vi "Neutral_voltage_conversions.vi"(8 "Constant":dbl, 9 "Final Value":dbl, 10 "Initial value":dbl, 11 "Conversion":T1=enum."B Field Grad (G/cm)") -> (1 "Final Voltage":dbl, 2 "Initial voltage":dbl)   [LabVIEW 2016]
uses:
  Neutral_voltage_conversion_control.ctl
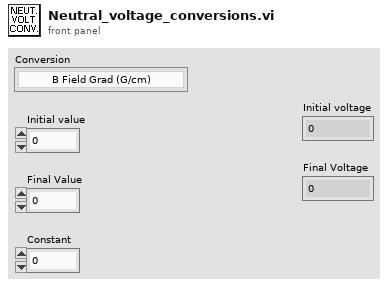
[diagram p1: front panel]
types:
  T1 = typedef "Neutral_voltage_conversion_control.ctl" = enum16{"Volts", "B Field Grad (G/cm)", "Red Boson Cntr Freq (MHz)", "Red Boson Dither Amp (kHz)", "Red Boson Power (mW)", "Red 87 Trap Cntr Freq (MHz)", "Red 87 Trap Dither Amp (kHz)", "Red 87 Trap Power (mW)", "Red 87 Stir Cntr Freq (MHz)", "Red 87 Stir Dither Amp (kHz)", "Red 87 Stir Power (mW)", "ODT Sheet Trap Power (W)", "ODT Loading Trap Power (W)"}
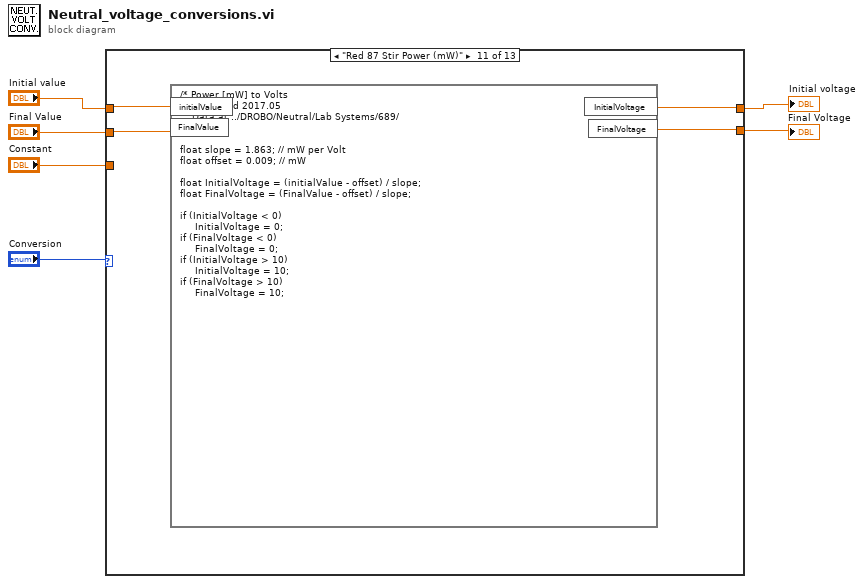
[diagram p0: block diagram]
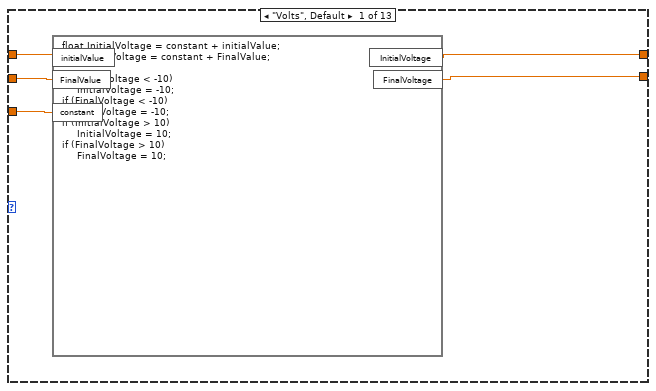
[diagram p2: hidden frame]
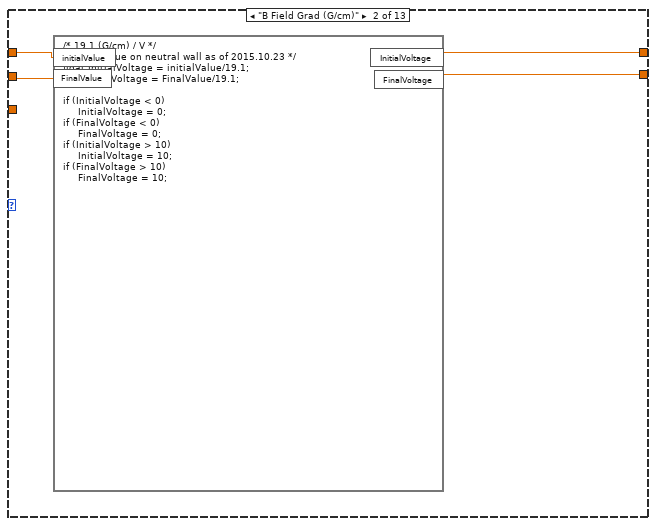
[diagram p3: hidden frame]
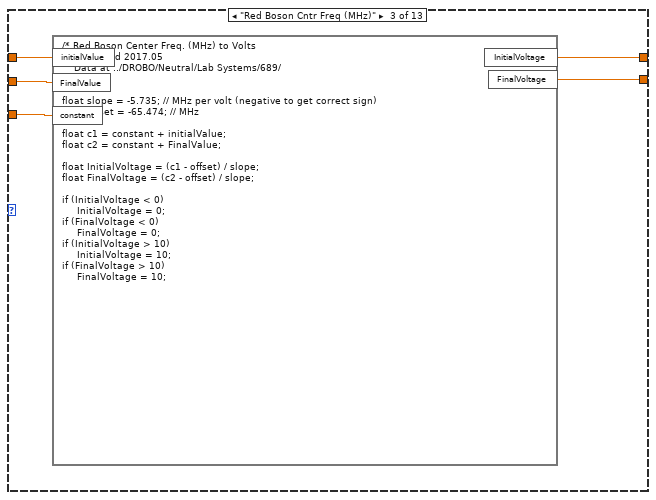
[diagram p4: hidden frame]
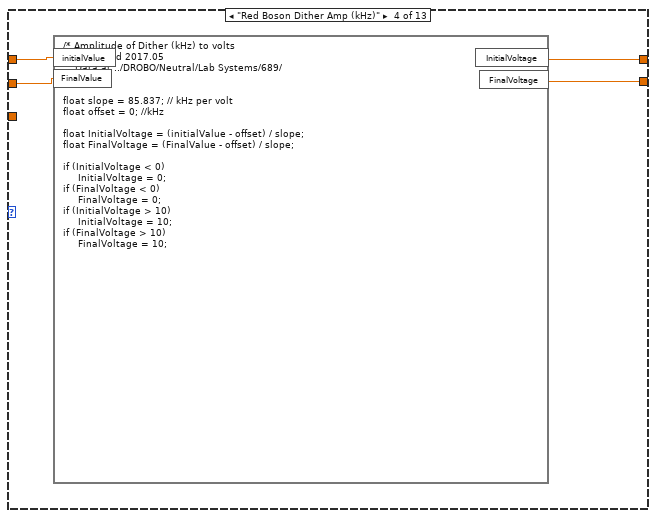
[diagram p5: hidden frame]
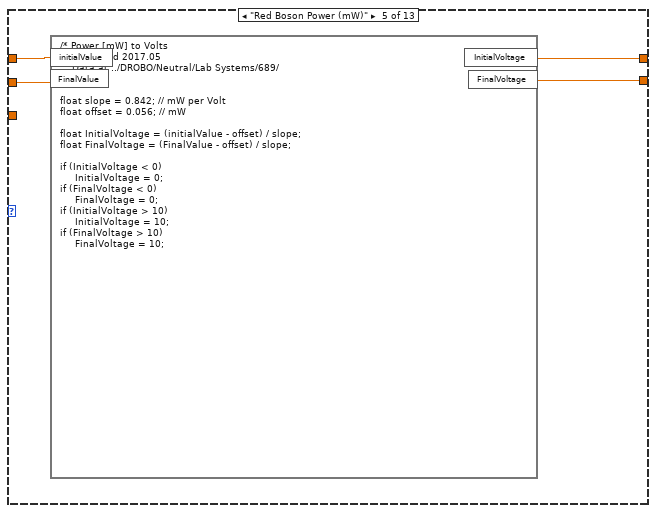
[diagram p6: hidden frame]
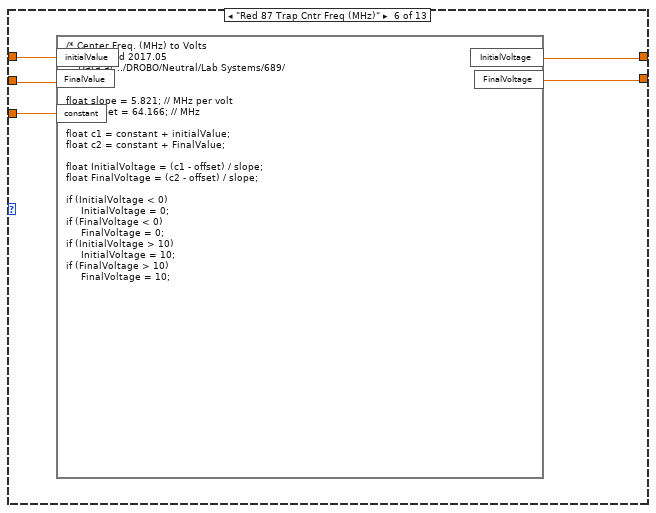
[diagram p7: hidden frame]
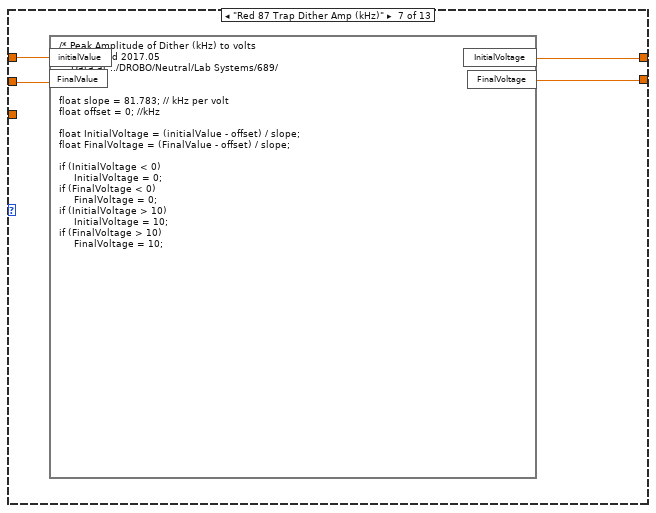
[diagram p8: hidden frame]
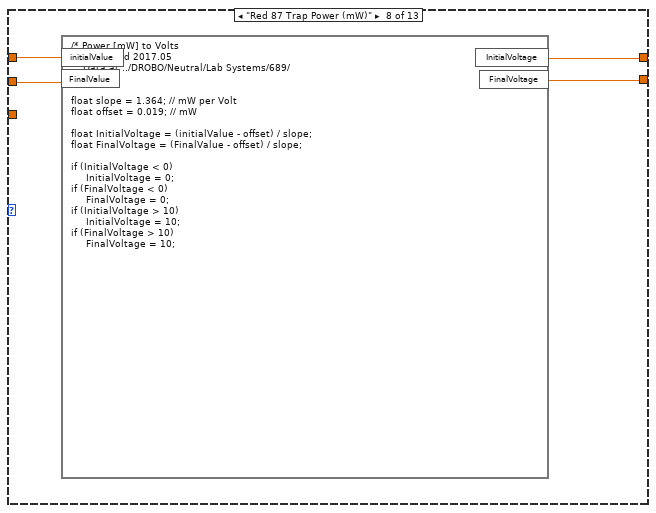
[diagram p9: hidden frame]
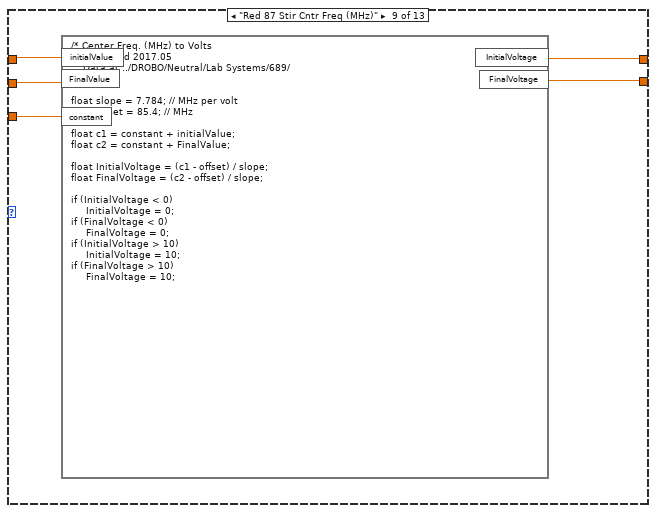
[diagram p10: hidden frame]
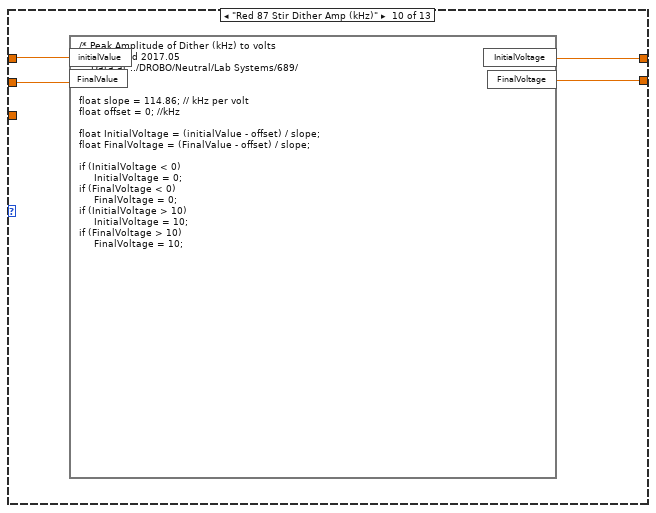
[diagram p11: hidden frame]
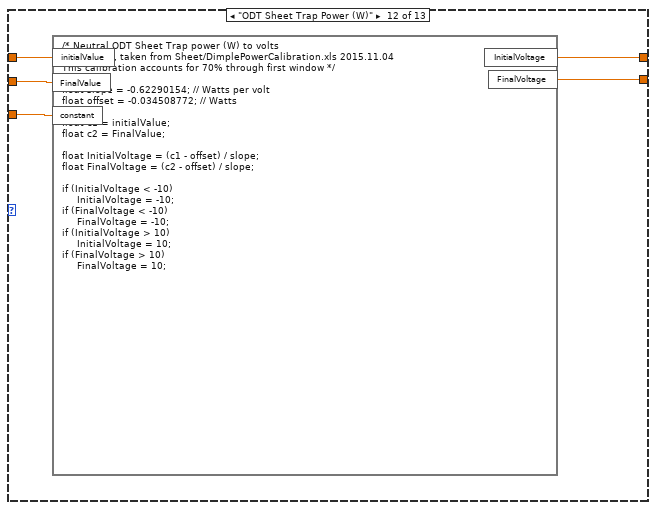
[diagram p12: hidden frame]
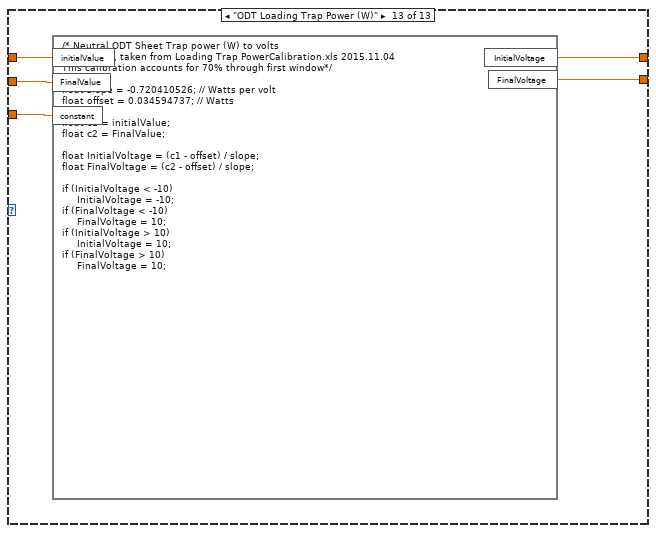
[diagram p13: hidden frame]
diagram:
  n1 = case shown="\"Red 87 Stir Power (mW)\"" "Conversion" {
    tunnel: "Initial value" -> [w9 w12 w20 w21 w28 w33 w35 w41 w46 w50 w54 w59 w64]
    tunnel: "Final Value" -> [w8 w13 w19 w22 w27 w32 w34 w40 w45 w49 w53 w58 w63]
    tunnel: [w10 w15 w18 w23 w25 w31 w36 w39 w43 w47 w52 w57 w62] -> w3
    tunnel: [w11 w14 w17 w24 w26 w30 w37 w38 w44 w48 w51 w56 w61] -> w2
    tunnel: "Constant" -> [w7 _ w16 _ _ w29 _ _ w42 _ _ w55 w60]
    frame "Volts", Default {
      n2 = formula code="float InitialVoltage = constant + initialValue;\nfloat FinalVoltage = constant + FinalValue;\n\nif (InitialVoltage < -10)\n     InitialVoltage = -10;\nif (FinalVoltage < -10)\n     FinalVoltage = -10;\nif (InitialVoltage > 10)\n     InitialVoltage = 10;\nif (FinalVoltage > 10)\n     FinalVoltage = 10;"("initialValue"=w9, "FinalValue"=w8, "constant"=w7) -> ("InitialVoltage"=w10:dbl, "FinalVoltage"=w11:dbl)
    }
    frame "B Field Grad (G/cm)" {
      n3 = formula code="/* 19.1 (G/cm) / V */\n/*Using value on neutral wall as of 2015.10.23 */\nfloat InitialVoltage = initialValue/19.1;\nfloat FinalVoltage = FinalValue/19.1;\n\nif (InitialVoltage < 0)\n     InitialVoltage = 0;\nif (FinalVoltage < 0)\n     FinalVoltage = 0;\nif (InitialVoltage > 10)\n     InitialVoltage = 10;\nif (FinalVoltage > 10)\n     FinalVoltage = 10;"("initialValue"=w12, "FinalValue"=w13) -> ("InitialVoltage"=w15:dbl, "FinalVoltage"=w14:dbl)
    }
    frame "Red Boson Cntr Freq (MHz)" {
      n4 = formula code="/* Red Boson Center Freq. (MHz) to Volts\n    Measured 2017.05\n    Data at ../DROBO/Neutral/Lab Systems/689/\n*/\n\nfloat slope = -5.735; // MHz per volt (negative to get correct sign)\nfloat offset = -65.474; // MHz\n\nfloat c1 = constant + initialValue;\nfloat c2 = constant + FinalValue;\n\nfloat InitialVoltage = (c1 - offset) / slope;\nfloat FinalVoltage = (c2 - offset) / slope;\n\nif (InitialVoltage < 0)\n     InitialVoltage = 0;\nif (FinalVoltage < 0)\n     FinalVoltage = 0;\nif (InitialVoltage > 10)\n     InitialVoltage = 10;\nif (FinalVoltage > 10)\n     FinalVoltage = 10;"("initialValue"=w20, "FinalValue"=w19, "constant"=w16) -> ("InitialVoltage"=w18:dbl, "FinalVoltage"=w17:dbl)
    }
    frame "Red Boson Dither Amp (kHz)" {
      n5 = formula code="/* Amplitude of Dither (kHz) to volts\n    Measured 2017.05\n    Data at ../DROBO/Neutral/Lab Systems/689/\n*/\n\nfloat slope = 85.837; // kHz per volt\nfloat offset = 0; //kHz\n\nfloat InitialVoltage = (initialValue - offset) / slope;\nfloat FinalVoltage = (FinalValue - offset) / slope;\n\nif (InitialVoltage < 0)\n     InitialVoltage = 0;\nif (FinalVoltage < 0)\n     FinalVoltage = 0;\nif (InitialVoltage > 10)\n     InitialVoltage = 10;\nif (FinalVoltage > 10)\n     FinalVoltage = 10;"("initialValue"=w21, "FinalValue"=w22) -> ("InitialVoltage"=w23:dbl, "FinalVoltage"=w24:dbl)
    }
    frame "Red Boson Power (mW)" {
      n6 = formula code="/* Power [mW] to Volts\n    Measured 2017.05\n    Data at ../DROBO/Neutral/Lab Systems/689/\n*/\n\nfloat slope = 0.842; // mW per Volt\nfloat offset = 0.056; // mW\n\nfloat InitialVoltage = (initialValue - offset) / slope;\nfloat FinalVoltage = (FinalValue - offset) / slope;\n\nif (InitialVoltage < 0)\n     InitialVoltage = 0;\nif (FinalVoltage < 0)\n     FinalVoltage = 0;\nif (InitialVoltage > 10)\n     InitialVoltage = 10;\nif (FinalVoltage > 10)\n     FinalVoltage = 10;"("initialValue"=w28, "FinalValue"=w27) -> ("InitialVoltage"=w25:dbl, "FinalVoltage"=w26:dbl)
    }
    frame "Red 87 Trap Cntr Freq (MHz)" {
      n7 = formula code="/* Center Freq. (MHz) to Volts\n    Measured 2017.05\n    Data at ../DROBO/Neutral/Lab Systems/689/\n*/\n\nfloat slope = 5.821; // MHz per volt\nfloat offset = 64.166; // MHz\n\nfloat c1 = constant + initialValue;\nfloat c2 = constant + FinalValue;\n\nfloat InitialVoltage = (c1 - offset) / slope;\nfloat FinalVoltage = (c2 - offset) / slope;\n\nif (InitialVoltage < 0)\n     InitialVoltage = 0;\nif (FinalVoltage < 0)\n     FinalVoltage = 0;\nif (InitialVoltage > 10)\n     InitialVoltage = 10;\nif (FinalVoltage > 10)\n     FinalVoltage = 10;"("initialValue"=w33, "FinalValue"=w32, "constant"=w29) -> ("InitialVoltage"=w31:dbl, "FinalVoltage"=w30:dbl)
    }
    frame "Red 87 Trap Dither Amp (kHz)" {
      n8 = formula code="/* Peak Amplitude of Dither (kHz) to volts\n    Measured 2017.05\n    Data at ../DROBO/Neutral/Lab Systems/689/\n*/\n\nfloat slope = 81.783; // kHz per volt\nfloat offset = 0; //kHz\n\nfloat InitialVoltage = (initialValue - offset) / slope;\nfloat FinalVoltage = (FinalValue - offset) / slope;\n\nif (InitialVoltage < 0)\n     InitialVoltage = 0;\nif (FinalVoltage < 0)\n     FinalVoltage = 0;\nif (InitialVoltage > 10)\n     InitialVoltage = 10;\nif (FinalVoltage > 10)\n     FinalVoltage = 10;"("initialValue"=w35, "FinalValue"=w34) -> ("InitialVoltage"=w36:dbl, "FinalVoltage"=w37:dbl)
    }
    frame "Red 87 Trap Power (mW)" {
      n9 = formula code="/* Power [mW] to Volts\n    Measured 2017.05\n    Data at ../DROBO/Neutral/Lab Systems/689/\n*/\n\nfloat slope = 1.364; // mW per Volt\nfloat offset = 0.019; // mW\n\nfloat InitialVoltage = (initialValue - offset) / slope;\nfloat FinalVoltage = (FinalValue - offset) / slope;\n\nif (InitialVoltage < 0)\n     InitialVoltage = 0;\nif (FinalVoltage < 0)\n     FinalVoltage = 0;\nif (InitialVoltage > 10)\n     InitialVoltage = 10;\nif (FinalVoltage > 10)\n     FinalVoltage = 10;"("initialValue"=w41, "FinalValue"=w40) -> ("InitialVoltage"=w39:dbl, "FinalVoltage"=w38:dbl)
    }
    frame "Red 87 Stir Cntr Freq (MHz)" {
      n10 = formula code="/* Center Freq. (MHz) to Volts\n    Measured 2017.05\n    Data at ../DROBO/Neutral/Lab Systems/689/\n*/\n\nfloat slope = 7.784; // MHz per volt\nfloat offset = 85.4; // MHz\n\nfloat c1 = constant + initialValue;\nfloat c2 = constant + FinalValue;\n\nfloat InitialVoltage = (c1 - offset) / slope;\nfloat FinalVoltage = (c2 - offset) / slope;\n\nif (InitialVoltage < 0)\n     InitialVoltage = 0;\nif (FinalVoltage < 0)\n     FinalVoltage = 0;\nif (InitialVoltage > 10)\n     InitialVoltage = 10;\nif (FinalVoltage > 10)\n     FinalVoltage = 10;"("initialValue"=w46, "FinalValue"=w45, "constant"=w42) -> ("InitialVoltage"=w43:dbl, "FinalVoltage"=w44:dbl)
    }
    frame "Red 87 Stir Dither Amp (kHz)" {
      n11 = formula code="/* Peak Amplitude of Dither (kHz) to volts\n    Measured 2017.05\n    Data at ../DROBO/Neutral/Lab Systems/689/\n*/\n\nfloat slope = 114.86; // kHz per volt\nfloat offset = 0; //kHz\n\nfloat InitialVoltage = (initialValue - offset) / slope;\nfloat FinalVoltage = (FinalValue - offset) / slope;\n\nif (InitialVoltage < 0)\n     InitialVoltage = 0;\nif (FinalVoltage < 0)\n     FinalVoltage = 0;\nif (InitialVoltage > 10)\n     InitialVoltage = 10;\nif (FinalVoltage > 10)\n     FinalVoltage = 10;"("initialValue"=w50, "FinalValue"=w49) -> ("InitialVoltage"=w47:dbl, "FinalVoltage"=w48:dbl)
    }
    frame "Red 87 Stir Power (mW)" {
      n12 = formula code="/* Power [mW] to Volts\n    Measured 2017.05\n    Data at ../DROBO/Neutral/Lab Systems/689/\n*/\n\nfloat slope = 1.863; // mW per Volt\nfloat offset = 0.009; // mW\n\nfloat InitialVoltage = (initialValue - offset) / slope;\nfloat FinalVoltage = (FinalValue - offset) / slope;\n\nif (InitialVoltage < 0)\n     InitialVoltage = 0;\nif (FinalVoltage < 0)\n     FinalVoltage = 0;\nif (InitialVoltage > 10)\n     InitialVoltage = 10;\nif (FinalVoltage > 10)\n     FinalVoltage = 10;"("initialValue"=w54, "FinalValue"=w53) -> ("InitialVoltage"=w52:dbl, "FinalVoltage"=w51:dbl)
    }
    frame "ODT Sheet Trap Power (W)" {
      n13 = formula code="/* Neutral ODT Sheet Trap power (W) to volts\ncalibration, taken from Sheet/DimplePowerCalibration.xls 2015.11.04\nThis calibration accounts for 70% through first window */\n\nfloat slope = -0.62290154; // Watts per volt\nfloat offset = -0.034508772; // Watts\n\nfloat c1 = initialValue;\nfloat c2 = FinalValue;\n\nfloat InitialVoltage = (c1 - offset) / slope;\nfloat FinalVoltage = (c2 - offset) / slope;\n\nif (InitialVoltage < -10)\n     InitialVoltage = -10;\nif (FinalVoltage < -10)\n     FinalVoltage = -10;\nif (InitialVoltage > 10)\n     InitialVoltage = 10;\nif (FinalVoltage > 10)\n     FinalVoltage = 10;"("initialValue"=w59, "FinalValue"=w58, "constant"=w55) -> ("InitialVoltage"=w57:dbl, "FinalVoltage"=w56:dbl)
    }
    frame "ODT Loading Trap Power (W)" {
      n14 = formula code="/* Neutral ODT Sheet Trap power (W) to volts\ncalibration, taken from Loading Trap PowerCalibration.xls 2015.11.04\nThis calibration accounts for 70% through first window*/\n\nfloat slope = -0.720410526; // Watts per volt\nfloat offset = 0.034594737; // Watts\n\nfloat c1 = initialValue;\nfloat c2 = FinalValue;\n\nfloat InitialVoltage = (c1 - offset) / slope;\nfloat FinalVoltage = (c2 - offset) / slope;\n\nif (InitialVoltage < -10)\n     InitialVoltage = -10;\nif (FinalVoltage < -10)\n     FinalVoltage = 10;\nif (InitialVoltage > 10)\n     InitialVoltage = 10;\nif (FinalVoltage > 10)\n     FinalVoltage = 10;"("initialValue"=w64, "FinalValue"=w63, "constant"=w60) -> ("InitialVoltage"=w62:dbl, "FinalVoltage"=w61:dbl)
    }
  }
  "Initial voltage" <- w3
  "Final Voltage" <- w2
